vi "Polygon to Point Array.vi"(8 "error in (no error)":errorcluster, 10 "Polygon Index":i32, 11 "Overlay Ref":refnum<k24>) -> (0 "error out":errorcluster, 3 "Points":refnum<k24>)   [LabVIEW 2014]
uses:
  C:/Robotic Systems/Products/AgFalcon/Software/Ground Station/Data/Mapping DLL/GMap.NET.WindowsForms.dll
  Data/Mapping DLL/GMap.NET.WindowsForms.dll
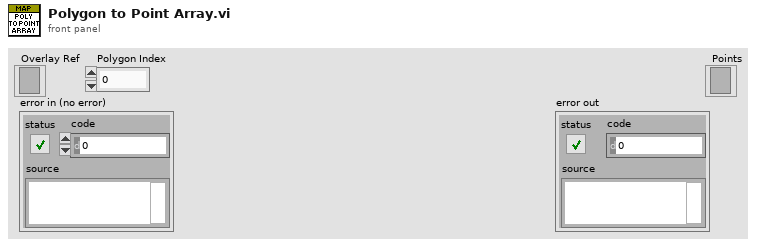
[diagram p1: front panel]
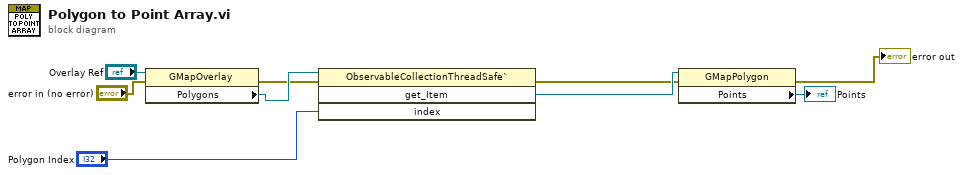
[diagram p0: block diagram]
diagram:
  n1 = property class="GMapOverlay"(reference="Overlay Ref", error in="error in (no error)") -> (error out=w6:errorcluster, "Polygons"=w7:refnum<k24>)  [unwired: 1 out]
  n2 = invoke class="ObservableCollectionThreadSafe`" method="get_Item"(reference=w7, error in=w6, "index"="Polygon Index") -> (error out=w3:errorcluster, "get_Item"=w4:refnum<k24>)  [unwired: 1 in, 2 out]
  n3 = property class="GMapPolygon"(reference=w4, error in=w3) -> (error out=→"error out":errorcluster, "Points"=→"Points":refnum<k24>)  [unwired: 1 out]
